vi "Bharat1.vi"() -> ()   [LabVIEW 2019]
uses:
  <vilib>/BLE/type_def/connection_status_bundle.ctl
  <vilib>/BLE/type_def/address_type.ctl
panel:
  out "Gradient graph":dbl(graph)
  out "Gradient":dbl
  out "Device Name":string
  out "Reading data":bool
  in  "stop":bool
  out "Connection Status":T1={"MAC Address"="", "cnx handle"=0, "cnx flags"=0, "Address Type"=125, "Connection Interval (ms)"=125, "Timeout(ms)"=125, "Latency"=0, "bonding handle"=0} {"Address Type" items=["Public", "Random"]}
  out "Connected":bool
  out "Handle table":string[][](array[string])
  out "Scanning":bool
  in  "COM Bluegiga in":refnum<visa-resource-name>="COM13"
  out "Devices":string[][](array[string])
  out "BLED112 Dongle Info":string
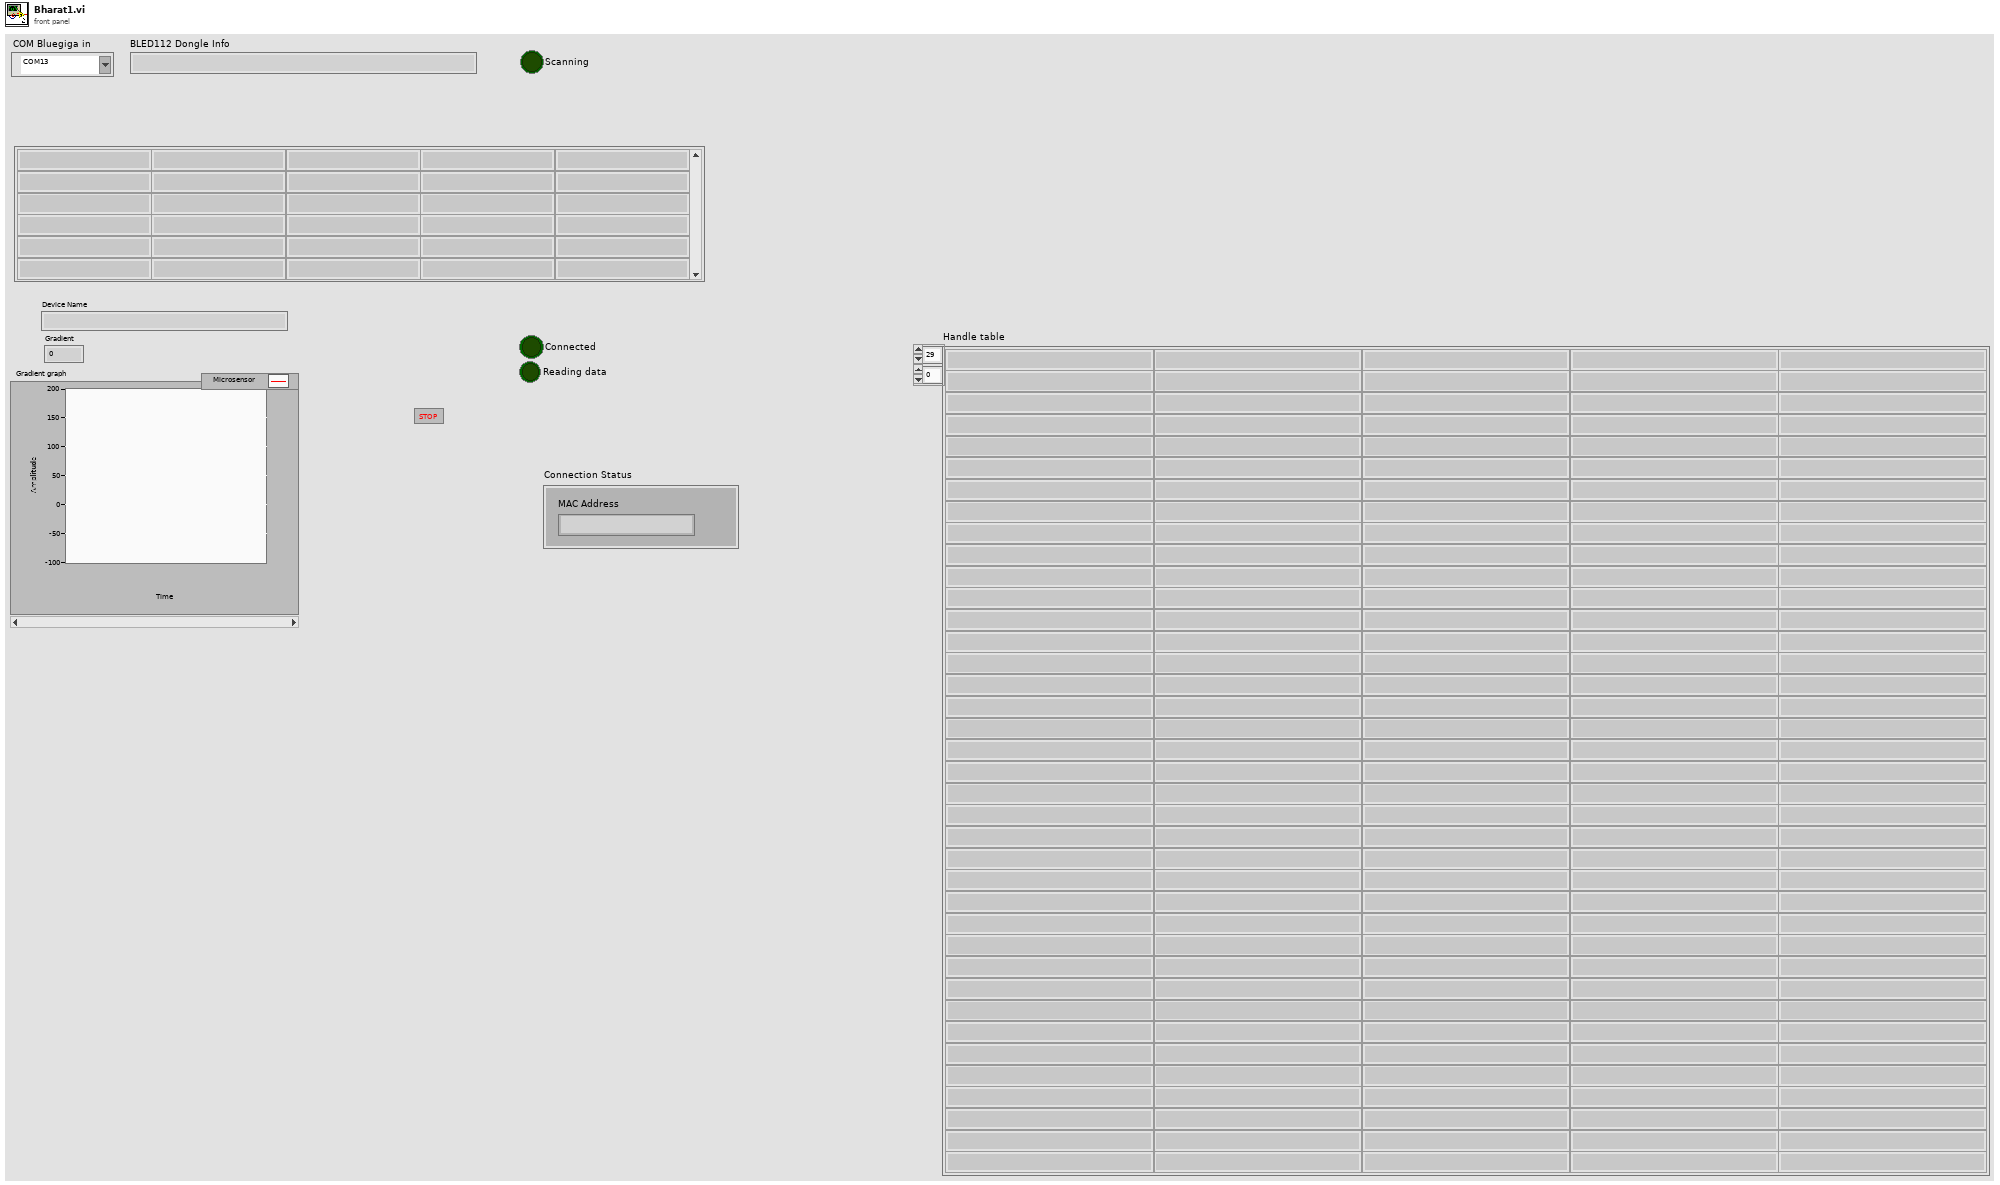
[diagram p1: front panel]
types:
  T1 = typedef "connection_status_bundle.ctl" = cluster{"MAC Address":string, "cnx handle":u8, "cnx flags":u8, "Address Type":T2, "Connection Interval (ms)":u16, "Timeout(ms)":u16, "Latency":u16, "bonding handle":u8}
  T2 = typedef "address_type.ctl" = u8
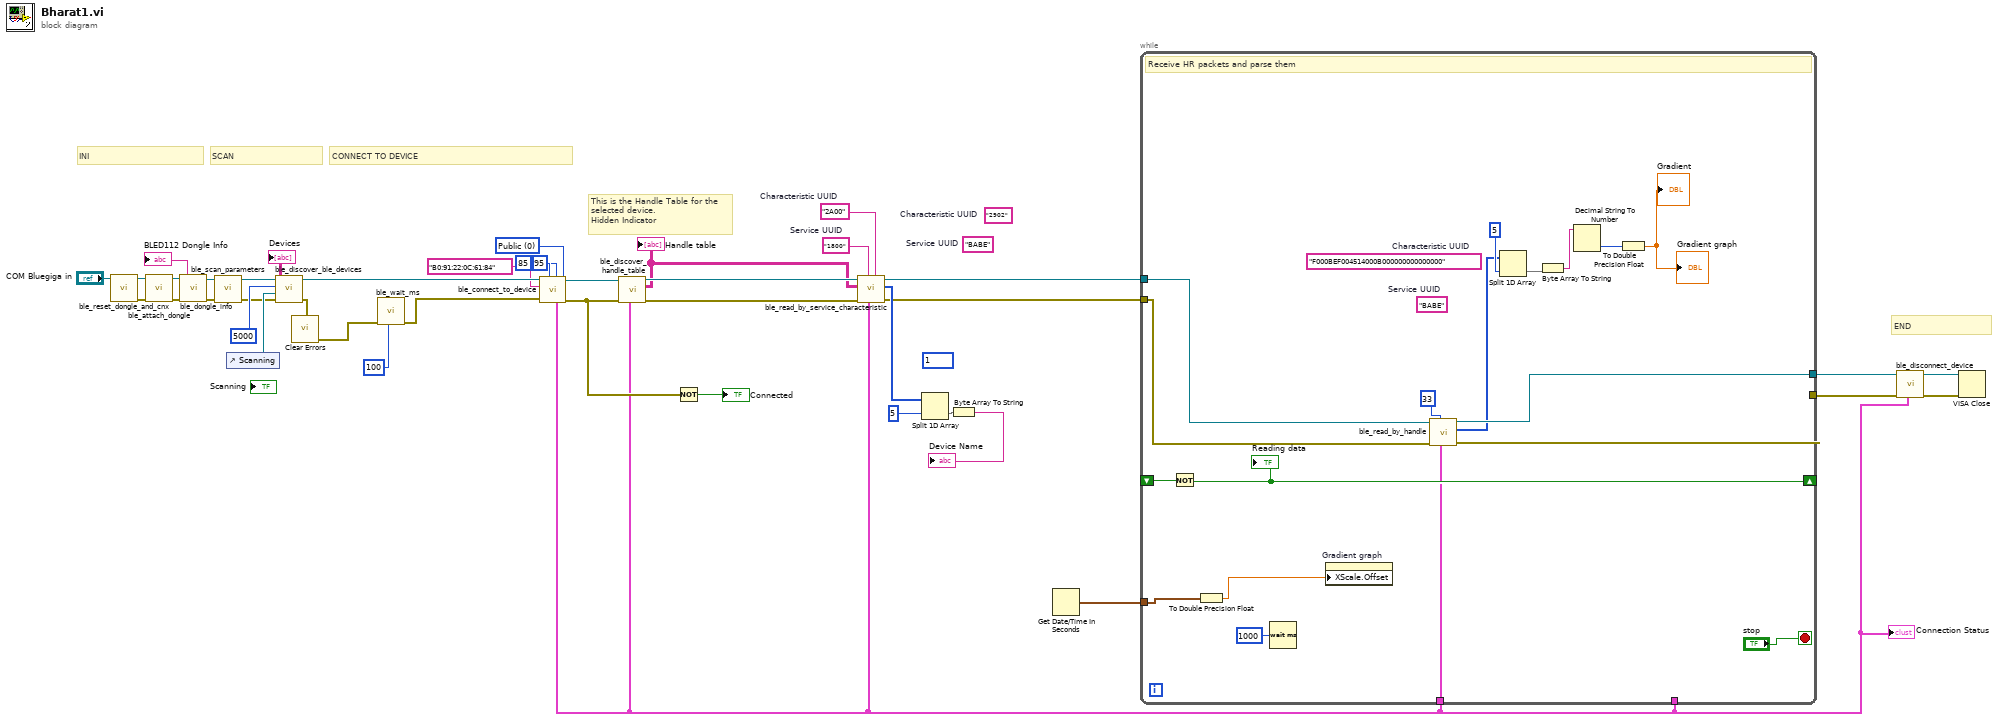
[diagram p0: block diagram]
diagram:
  w17 = T2 0 items=["Public", "Random"] ("Address Type")
  (unwired) "2902"  # Characteristic UUID
  (unwired) "BABE"  # Service UUID
  (unwired) u16 1 ("Value(16bit)")
  w22 = "2A00"  # Characteristic UUID
  w23 = "1800"  # Service UUID
  # "END"
  # "This is the Handle Table for the\nselected device. \nHidden Indicator"
  # "CONNECT TO DEVICE"
  # "SCAN"
  # "INI"
  n1 = call <vilib>:"ble_reset_dongle_and_cnx.vi"("COM Bluegiga in"="COM Bluegiga in") -> ("error out"=w32:errorcluster, "COM Bluegiga out"=w30:refnum<visa-resource-name>)  [unwired: 9 in]
  n2 = call <vilib>:"ble_attach_dongle.vi"("error in (no error)"=w32, "COM Bluegiga in"=w30) -> ("error out"=w34:errorcluster, "COM Bluegiga out"=w33:refnum<visa-resource-name>)  [unwired: 8 in]
  n3 = call <vilib>:"ble_dongle_info.vi"("error in (no error)"=w34, "COM Bluegiga in"=w33) -> ("error out"=w37:errorcluster, "info"=→"BLED112 Dongle Info":string, "COM Bluegiga out"=w38:refnum<visa-resource-name>)  [unwired: 7 in]
  n4 = call <vilib>:"ble_scan_parameters.vi"("error in (no error)"=w37, "COM Bluegiga in"=w38) -> ("error out"=w35:errorcluster, "COM Bluegiga out"=w36:refnum<visa-resource-name>)  [unwired: 7 in, 1 out]
  n5 = control-ref of="Scanning"() -> (w39:refnum<vi>)
  n6 = call <vilib>:"ble_discover_ble_devices.vi"("error in (no error)"=w35, "LED ref"=w39, "Scan Duration (10000ms)"=u32 5000, "COM Bluegiga in"=w36) -> ("error out"=w28:errorcluster, "Devices"=→"Devices":string[][], "COM Bluegiga out"=w18:refnum<visa-resource-name>)  [unwired: 5 in]
  n7 = call <vilib>:"Clear Errors.vi"("error in (no error)"=w28) -> ("error out"=w21:errorcluster)  [unwired: 5 in, 1 out]
  n8 = call <vilib>:"ble_wait_ms.vi"("milliseconds to wait (100)"=u32 100, "error in (no error)"=w21) -> ("error out"=w20:errorcluster)  [unwired: 9 in]
  n9 = call <vilib>:"ble_connect_to_device.vi"("Address Type"=w17, "Connection Interval Max (95ms)"=u16 95, "Connection Interval Min (75ms)"=u16 85, "error in (no error)"=w20, "MAC Address"="B0:91:22:0C:61:84", "COM Bluegiga in"=w18) -> ("error out"=w24:errorcluster, "COM Bluegiga out"=w29:refnum<visa-resource-name>, "Connection Status"=w5:T1)  [unwired: 3 in]
  "Connection Status" <- w5
  n10 = call <vilib>:"ble_discover_handle_table.vi"("Connection Status"=w5, "error in (no error)"=w24, "COM Bluegiga in"=w29) -> ("error out"=w27:errorcluster, "Handle table"=w11:string[][], "COM Bluegiga out"=w26:refnum<visa-resource-name>)  [unwired: 6 in]
  "Handle table" <- w11
  n11 = Not(x=w24) -> (.not. x?=→"Connected":bool)
  n12 = call <vilib>:"ble_read_by_service_characteristic.vi"("Characteristic UUID"=w22, "Connection Status"=w5, "Service UUID"=w23, "error in (no error)"=w27, "Handle table"=w11, "COM Bluegiga in"=w26) -> ("error out"=w1:errorcluster, "characteristic value"=w6:u8[], "COM Bluegiga out"=w2:refnum<visa-resource-name>)  [unwired: 3 in]
  n13 = Split 1D Array(array=w6, index=5) -> (second subarray=w7:u8[])  [unwired: 1 out]
  n14 = Byte Array To String(unsigned byte array=w7) -> (string=→"Device Name":string)
  n15 = Get Date/Time In Seconds() -> (seconds since 1Jan1904=w10:timestamp)
  n16 = while {
    shift-right: [w57] -> _
    shift-left: _ -> [w56]
    tunnel: w5 -> [_]
    tunnel: w10 -> [w58]
    tunnel: w5 -> [w48]
    tunnel: [w45] -> w4
    tunnel: [w44] -> w3
    tunnel: w2 -> [w47]
    tunnel: w1 -> [w46]
    stop <- "stop" stop-if-true
    (unwired) "F000BEF004514000B000000000000000"  # Characteristic UUID
    (unwired) "BABE"  # Service UUID
    # "Receive HR packets and parse them"
    n17 = Not(x=w56) -> (.not. x?=w57:bool)
    "Reading data" <- w57
    n18 = To Double Precision Float(number=w58) -> (double precision float=w49:dbl)
    n19 = Wait (ms)(milliseconds to wait=u32 1000) -> ()  [unwired: 1 out]
    n20 = property on="Gradient graph" class="WFChart (strict)"("XScale.Offset"=w49) -> ()  [unwired: 2 in, 2 out]
    n21 = call <vilib>:"ble_read_by_handle.vi"("Connection Status"=w48, "Handle"=u16 33, "error in (no error)"=w46, "COM Bluegiga in"=w47) -> ("error out"=w44:errorcluster, "characteristic value"=w43:u8[], "COM Bluegiga out"=w45:refnum<visa-resource-name>)  [unwired: 5 in]
    n22 = Split 1D Array(array=w43, index=5) -> (second subarray=w54:u8[])  [unwired: 1 out]
    n23 = Byte Array To String(unsigned byte array=w54) -> (string=w53:string)
    n24 = Decimal String To Number(string=w53) -> (number=w52:i32)  [unwired: 2 in, 1 out]
    n25 = To Double Precision Float(number=w52) -> (double precision float=→"Gradient" →"Gradient graph":dbl)
  }
  n26 = call <vilib>:"ble_disconnect_device.vi"("Connection Status"=w5, "error in (no error)"=w3, "COM Bluegiga in"=w4) -> ("error out"=w12:errorcluster, "COM Bluegiga out"=w13:refnum<visa-resource-name>)  [unwired: 7 in]
  n27 = VISA Close(VISA resource name=w13, error in (no error)=w12) -> ()  [unwired: 1 out]
